vi "MGI Executable Checksum.vi"() -> (0 "Checksum":u32)   [LabVIEW 2016]
doc: "Compute the checksum of the .exe file if an executable is running. FFFFFFFF is returned when running from the development system.\n\nAuthored by David A. Moore\nsupport@mooregoodideas.com\nwww.mooregoodideas.com\n\nCopyright (c) 2010, Moore Good Ideas, Inc.\n\nAll rights reserved.\n\nRedistribution and use in source and binary forms, with or without modification, are permitted provided that the following conditions are met:\n\n * Redistributions of source code must retain the above copyright notice, this list of conditions and the following disclaimer.\n * Redistributions in binary form must reproduce the above copyright notice, this list of conditions and the following disclaimer in the documentation and/or other materials provided with the distribution.\n * Neither the name of Moore Good Ideas, Inc. nor the names of its contributors may be used to endorse or promote products derived from this software without specific prior written permission.\n\nTHIS SOFTWARE IS PROVIDED BY THE COPYRIGHT HOLDERS AND CONTRIBUTORS \"AS IS\" AND ANY EXPRESS OR IMPLIED WARRANTIES, INCLUDING, BUT NOT LIMITED TO, THE IMPLIED WARRANTIES OF MERCHANTABILITY AND FITNESS FOR A PARTICULAR PURPOSE ARE DISCLAIMED. IN NO EVENT SHALL THE COPYRIGHT OWNER OR CONTRIBUTORS BE LIABLE FOR ANY DIRECT, INDIRECT, INCIDENTAL, SPECIAL, EXEMPLARY, OR CONSEQUENTIAL DAMAGES (INCLUDING, BUT NOT LIMITED TO, PROCUREMENT OF SUBSTITUTE GOODS OR SERVICES; LOSS OF USE, DATA, OR PROFITS; OR BUSINESS INTERRUPTION) HOWEVER CAUSED AND ON ANY THEORY OF LIABILITY, WHETHER IN CONTRACT, STRICT LIABILITY, OR TORT (INCLUDING NEGLIGENCE OR OTHERWISE) ARISING IN ANY WAY OUT OF THE USE OF THIS SOFTWARE, EVEN IF ADVISED OF THE POSSIBILITY OF SUCH DAMAGE."
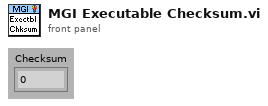
[diagram p1: front panel]
types:
  T1 = enum32{"invalid app kind", "Development System", "Run Time System", "Student Edition", "Embedded LabVIEW", "Evaluation", "Custom"}
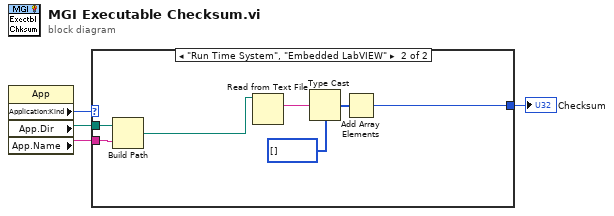
[diagram p0: block diagram]
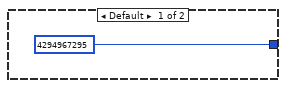
[diagram p2: hidden frame]
diagram:
  n1 = property class="App"() -> ("Application:Kind"=w4:T1, "App.Dir"=w2:path, "App.Name"=w1:string)  [unwired: 2 in, 2 out]
  n2 = case shown="\"Run Time System\", \"Embedded LabVIEW\"" w4 {
    tunnel: [u32 4294967295 w10] -> w3
    tunnel: w2 -> [_ w8]
    tunnel: w1 -> [_ w7]
    frame Default {
    }
    frame "Run Time System", "Embedded LabVIEW" {
      n3 = Build Path(base path=w8, name or relative path=w7) -> (appended path=w6:path)
      n4 = Read from Text File(file (use dialog)=w6) -> (text=w9:string)  [unwired: 3 in, 3 out]
      n5 = Type Cast(type=u32[] [], x=w9) -> (*(type *) &x=w11:u32[])
      n6 = Add Array Elements(numeric array=w11) -> (sum=w10:u32)
    }
  }
  "Checksum" <- w3
